vi "Get Config Path.vi"(8 "error in (no error)":errorcluster, 9 "section":string, 10 "key":string, 11 "Output Actor Hardware in":refnum<class "Output Actor Hardware.lvclass">) -> (0 "error out":errorcluster, 1 "found?":bool, 2 "value":bool, 3 "Output Actor Hardware out":refnum<class "Output Actor Hardware.lvclass">)   [LabVIEW 2015, in "Output Actor Hardware.lvclass"]
uses:
  Output Actor Hardware.lvclass
  Output Actor Hardware Interface/Output Actor Hardware Interface.lvclass
  Output Actor Hardware Interface/Get Config Value Bool.vi
  Output Actor/Output Actor.lvclass
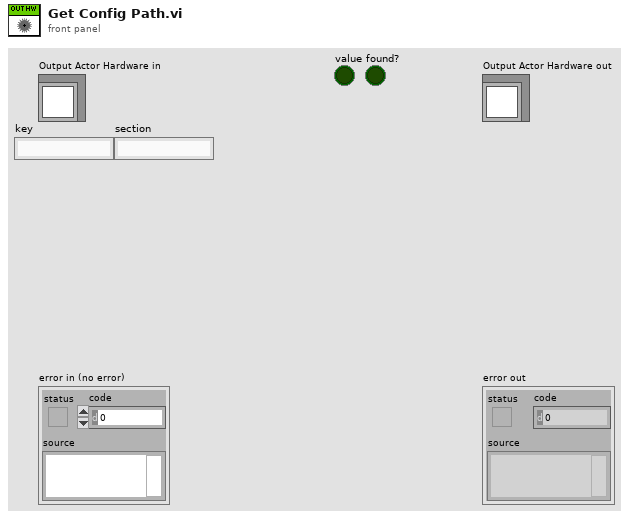
[diagram p1: front panel]
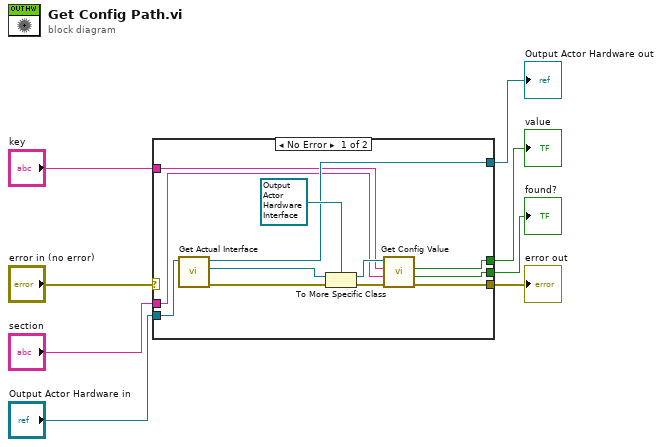
[diagram p0: block diagram]
diagram:
  n1 = case shown="No Error" "error in (no error)" {
    selector: "error in (no error)" -> [_ w22]
    tunnel: [w13 w22] -> w7
    tunnel: [w14 w21] -> w5
    tunnel: "Output Actor Hardware in" -> [w20 w21]
    tunnel: "section" -> [w12 _]
    tunnel: "key" -> [w11 _]
    tunnel: [w10 _] -> w2
    tunnel: [w9 _] -> w1
    frame No Error {
      n2 = call "Get Actual Interface.vi"("Output Actor in"=w20) -> ("error out"=w16:errorcluster, "Interface"=w19:refnum<class "Output Actor Interface.lvclass">, "Output Actor out"=w14:refnum<class "Output Actor Hardware.lvclass">)  [unwired: 8 in]
      n3 = To More Specific Class(target class=refnum<class "Output Actor Hardware Interface.lvclass"> refnum ("Output Actor Hardware Interface.lvclass"), reference=w19, error in=w16) -> (specific class reference=w17:refnum<class "Output Actor Hardware Interface.lvclass">, error out=w15:errorcluster)
      n4 = call-poly "Get Config Value.vi"("error in (no error)"=w15, "section"=w12, "key"=w11, "Output Actor Hardware Interface.lvclass"=w17) -> ("error out"=w13:errorcluster, "found?"=w9:bool, "value"=w10:bool)  [unwired: 4 in, 1 out]
    }
    frame Error {
    }
  }
  "error out" <- w7
  "Output Actor Hardware out" <- w5
  "value" <- w2
  "found?" <- w1
